vi "Waiting Pulse.vi"(8 "error in (no error)":errorcluster, 11 "Channel GUI in":refnum<class "Channel GUI.lvclass">) -> (0 "error out":errorcluster, 2 "waiting pulse ?":bool, 3 "Channel GUI out":refnum<class "Channel GUI.lvclass">)   [LabVIEW 2018, in "Channel GUI.lvclass"]
uses:
  Channel GUI.lvclass
  Channel GUI.lvclass/Channel GUI.ctl
  Stream/Stream.lvclass
  Interface/Interface.lvclass
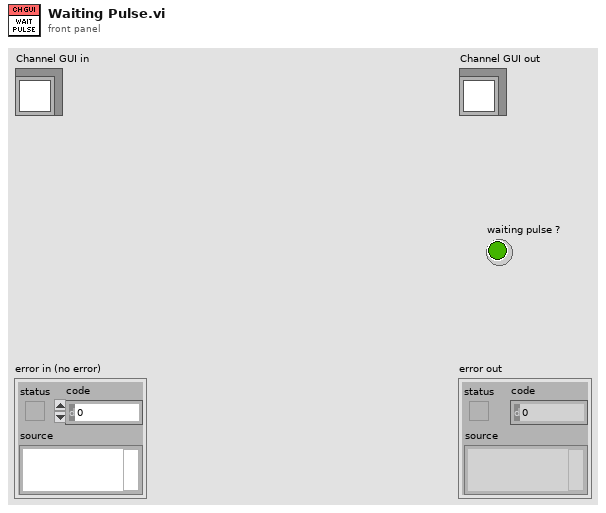
[diagram p1: front panel]
types:
  T1 = cluster{"% Acquired":u16, "Acquiring":bool, "Current image name":string, "Current sequence":u16, "CCD State":string}
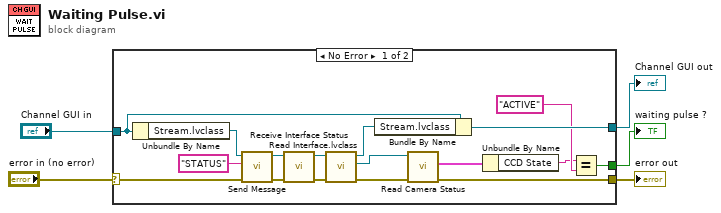
[diagram p0: block diagram]
diagram:
  n1 = case shown="No Error" "error in (no error)" {
    selector: "error in (no error)" -> [w17 w24]
    tunnel: [w20 w24] -> w4
    tunnel: [w21 w23] -> w2
    tunnel: "Channel GUI in" -> [w22 w23]
    tunnel: [w18 _] -> w1
    frame No Error {
      n2 = Unbundle By Name(w22) -> ("Stream.lvclass"=w16:refnum<class "Stream.lvclass">)
      n3 = call "Send Message.vi"("error in (no error)"=w17, "Message"="STATUS", "Stream in"=w16) -> ("error out"=w6:errorcluster, "Stream out"=w7:refnum<class "Stream.lvclass">)  [unwired: 7 in]
      n4 = call "Receive Interface Status.vi"("error in (no error)"=w6, "Stream in"=w7) -> ("error out"=w10:errorcluster, "Stream out"=w11:refnum<class "Stream.lvclass">)  [unwired: 8 in]
      n5 = call "Read Interface.lvclass.vi"("error in (no error)"=w10, "Stream in"=w11) -> ("error out"=w13:errorcluster, "Interface.lvclass"=w14:refnum<class "Interface.lvclass">, "Stream out"=w19:refnum<class "Stream.lvclass">)  [unwired: 7 in]
      n6 = Bundle By Name(cluster=w22, "Stream.lvclass"=w19) -> (w21:refnum<class "Channel GUI.lvclass">)
      n7 = call "Read Camera Status.vi"("error in (no error)"=w13, "Interface in"=w14) -> ("error out"=w20:errorcluster, "Camera Status"=w15:T1)  [unwired: 7 in, 1 out]
      n8 = Unbundle By Name(w15) -> ("CCD State"=w9:string)
      n9 = Equal?(x=w9, y="ACTIVE") -> (x = y?=w18:bool)
    }
    frame Error {
    }
  }
  "error out" <- w4
  "Channel GUI out" <- w2
  "waiting pulse ?" <- w1
